vi "Move_Off_Particles.vi"(4 "SD":dbl=1.0, 8 "Center State at T":T1, 9 "Ini_Anchor_Posi":dbl[][](array[numeric]), 11 "Particle Posi at T":T3(array[cluster])) -> (0 "Center State at T":T1, 3 "New Particle Posi at T":T2(array[cluster]))   [LabVIEW 2020]
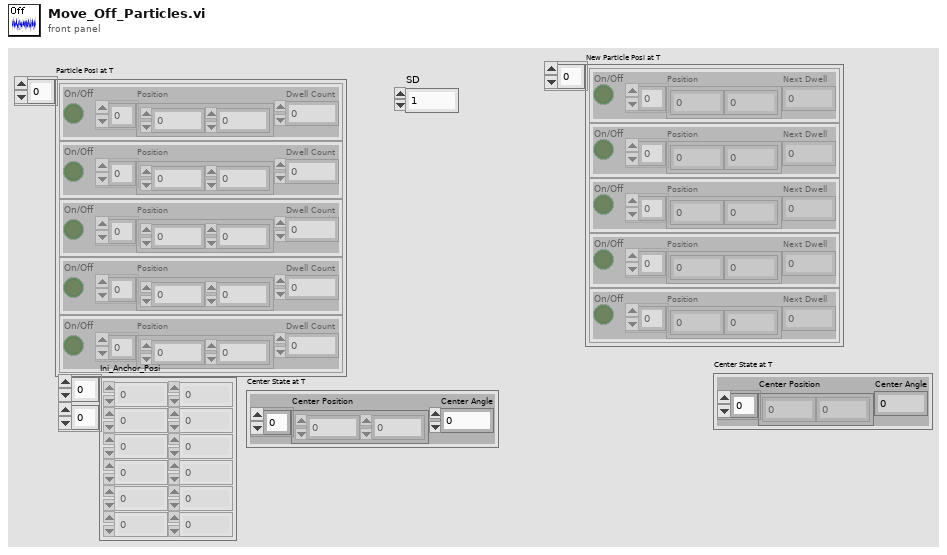
[diagram p1: front panel]
types:
  T1 = cluster{"Center Position":dbl[], "Center Angle":dbl}
  T2 = cluster{"On/Off":bool, "Position":dbl[], "Next Dwell":i32}[]
  T3 = cluster{"On/Off":bool, "Position":dbl[], "Dwell Count":i32}[]
  T4 = cluster{bool, "Position":dbl[], "Dwell Count":i32}
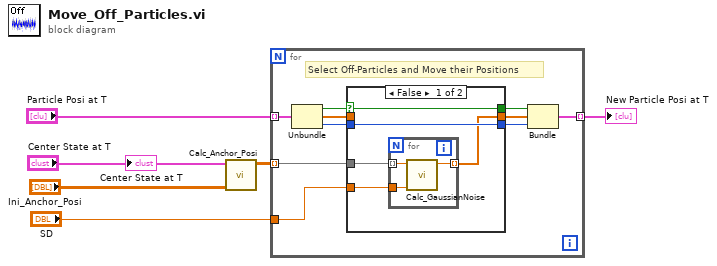
[diagram p0: block diagram]
diagram:
  n1 = call "Calc_Anchor_Posi.vi"("Initial Anchor Position"="Ini_Anchor_Posi", "Center State at T"="Center State at T") -> ("Anchor Posi at T"=w3:dbl[][])  [unwired: 9 in]
  n2 = for {
    tunnel: "Particle Posi at T" -> [w16] mode=indexing
    tunnel: [w15] -> w5 mode=indexing
    tunnel: "SD" -> [w8]
    tunnel: w3 -> [w7] mode=indexing
    # "Select Off-Particles and Move their Positions"
    n3 = Unbundle(w16) -> ("On/Off"=w14:bool, "Position"=w12:dbl[], "Dwell Count"=w10:i32)
    n4 = case shown="FALSE" w14 {
      selector: w14 -> [w21 w27]
      tunnel: [w21 w27] -> w13
      tunnel: [w18 w25] -> w11
      tunnel: w12 -> [_ w25]
      tunnel: [w20 w26] -> w9
      tunnel: w10 -> [w20 w26]
      tunnel: w8 -> [w19 _]
      tunnel: w7 -> [w17 _]
      frame False {
        n5 = for {
          tunnel: w17 -> [w24] mode=indexing
          tunnel: w19 -> [w23]
          tunnel: [w22] -> w18 mode=indexing
          n6 = call "Calc_GaussianNoise.vi"("SD"=w23, "Start Position"=w24) -> ("Final Position"=w22:dbl)  [unwired: 9 in]
        }
      }
      frame True {
      }
    }
    n7 = Bundle(w13, "Position"=w11, "Dwell Count"=w9) -> (w15:T4)  [unwired: 1 in]
  }
  "New Particle Posi at T" <- w5
  "Center State at T" <- "Center State at T"
